vi "RemoveZeroAmp.vi"(7 "Complex Waveform In":T3 {"y" format="%.2f"; "dx" format="%^.2e"; "x0" format="%^.2e"}) -> (8 "Real Waveform out":T1 {"y" min=0 max=127 format="%.2f"; "dx" format="%^.2e"; "x0" format="%^.2e"})   [LabVIEW 2016]
uses:
  niRFUtil/Includes/niRFUtil INC Complex Waveform.ctl
  niRFUtil/Includes/niRFUtil INC Complex Array.ctl
  niRFUtil/Includes/niRFUtil INC Real Waveform.ctl
  niRFUtil/Includes/niRFUtil INC Real Array.ctl
  niRFUtil/niRFUtil.lvlib
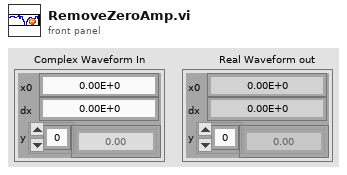
[diagram p1: front panel]
types:
  T1 = typedef "niRFUtil.lvlib/niRFUtil INC Real Waveform.ctl" = cluster{"x0":dbl, "dx":dbl, "y":T2}
  T2 = typedef "niRFUtil.lvlib/niRFUtil INC Real Array.ctl" = sgl[]
  T3 = typedef "niRFUtil.lvlib/niRFUtil INC Complex Waveform.ctl" = cluster{"x0":dbl, "dx":dbl, "y":T4}
  T4 = typedef "niRFUtil.lvlib/niRFUtil INC Complex Array.ctl" = csg[]
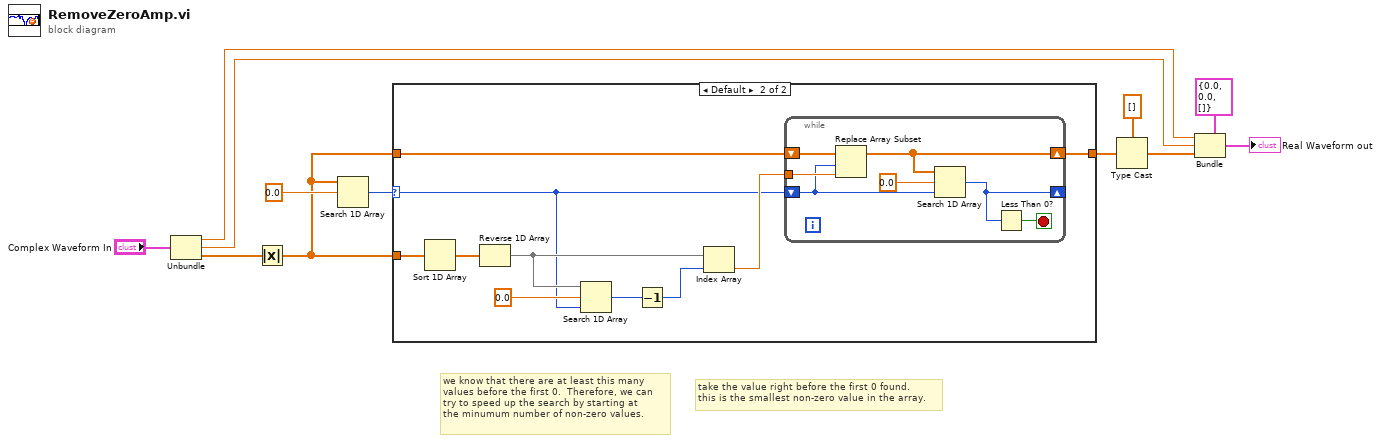
[diagram p0: block diagram]
diagram:
  # "take the value right before the first 0 found.\nthis is the smallest non-zero value in the array."
  # "we know that there are at least this many\nvalues before the first 0.  Therefore, we can\ntry to speed up the search by starting at\nthe minumum number of non-zero values."
  n1 = Unbundle("Complex Waveform In") -> ("x0"=w7:dbl, "dx"=w8:dbl, "y"=w10:T4)
  n2 = Absolute Value(x=w10) -> (abs(x)=w9:sgl[])
  n3 = Search 1D Array(1D array=w9, element=sgl 0.0) -> (index of element=w12:i32)  [unwired: 1 in]
  n4 = case shown="Default" w12 {
    selector: w12 -> [_ w15]
    tunnel: [w13 w19] -> w6
    tunnel: w9 -> [_ w17]
    tunnel: w9 -> [w13 w14]
    frame -1 {
    }
    frame Default {
      n5 = Sort 1D Array(array=w17) -> (sorted array=w23:sgl[])
      n6 = Reverse 1D Array(array=w23) -> (reversed array=w18:sgl[])
      n7 = Search 1D Array(1D array=w18, element=sgl 0.0, start index (0)=w15) -> (index of element=w22:i32)
      n8 = Decrement(x=w22) -> (x-1=w21:i32)
      n9 = Index Array(array=w18, index=w21) -> (element=w20:sgl)
      n10 = while {
        tunnel: w20 -> [w29]
        shift-right: [w26] -> w19
        shift-left: w14 -> [w30]
        shift-right: [w25] -> _
        shift-left: w15 -> [w28]
        stop <- w24 stop-if-true
        n11 = Replace Array Subset(array=w30, new element=w29, index=w28) -> (w26:sgl[])
        n12 = Search 1D Array(1D array=w26, element=sgl 0.0, start index (0)=w28) -> (index of element=w25:i32)
        n13 = Less Than 0?(x=w25) -> (x < 0?=w24:bool)
      }
    }
  }
  n14 = Type Cast(type=T2 [] ("y"), x=w6) -> (*(type *) &x=w3:T2)
  n15 = Bundle(cluster=T1 {"x0"=0.0, "dx"=0.0, "y"=[]} ("Real Waveform out 2"), "x0"=w7, "dx"=w8, "y"=w3) -> (→"Real Waveform out":T1)
